vi "PostToWatson.vi"(9 "Model Name":string="default", 11 "image in":T1) -> (0 "All Data":T2, 1 "Most likely":cluster{"score":dbl, "class":string}[](array[cluster]), 2 "class":string, 3 "image out":T1, 4 "score":dbl)   [LabVIEW 2019]
uses:
  <vilib>/picture/picture.llb/imagedata.ctl
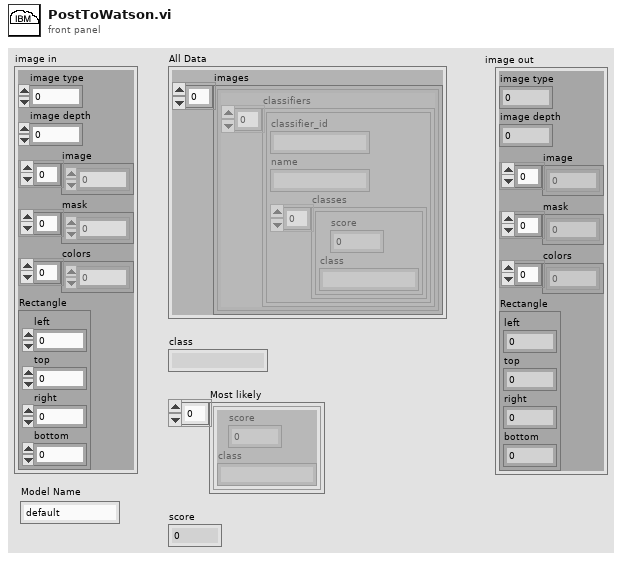
[diagram p1: front panel]
types:
  T1 = typedef "imagedata.ctl" = cluster{"image type":i32, "image depth":i32, "image":u8[], "mask":u8[], "colors":u32[], "Rectangle":cluster{"left":i16, "top":i16, "right":i16, "bottom":i16}}
  T2 = cluster{"images":cluster{"classifiers":cluster{"classifier_id":string, "name":string, "classes":cluster{"score":dbl, "class":string}[]}[]}[]}
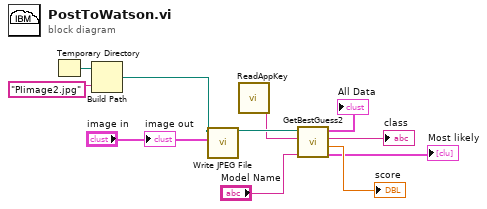
[diagram p0: block diagram]
diagram:
  n1 = Temporary Directory() -> (w6:path)
  n2 = Build Path(base path=w6, name or relative path="PIimage2.jpg") -> (appended path=w8:path)
  n3 = call <vilib>:"Write JPEG File.vi"("image data"="image in", "path to JPEG file"=w8) -> ("path"=w4:path)  [unwired: 8 in, 1 out]
  n4 = call "ReadAppKey.vi"() -> ("APIKey"=w3:string)  [unwired: 11 in]
  n5 = call "GetBestGuess2.vi"("Classifier"="Model Name", "APIKey"=w3, "Image"=w4) -> ("Most likely"=→"Most likely":cluster{"score":dbl, "class":string}[], "score"=→"score":dbl, "class"=→"class":string, "All Data"=→"All Data":T2)  [unwired: 5 in]
  "image out" <- "image in"
